vi "sharp_ir_long.vi"(11 "ana_volts":dbl) -> (3 "eng_cm":dbl)   [LabVIEW 2012]
panel:
  in  "cm":dbl[](array[numeric])=[200.0, 150.0, 140.0, 130.0, 120.0, 110.0, 100.0, 90.0, 80.0, 70.0, 60.0, 50.0, 40.0, 30.0, 20.0, 15.0, 0.0]
  in  "volts":dbl[](array[numeric])=[0.0, 0.4, 0.45, 0.5, 0.55, 0.6, 0.66, 0.73, 0.8, 0.86, 1.07, 1.25, 1.56, 2.0, 2.5, 2.75, 5.0]
  # "This function is a transfer function for the Sharp IR GP2Y0A02YK0F long range IR rangefinder\nThis curve is copied directly from the Sharp spec sheet transfer curve. Units are cm in that sheet."
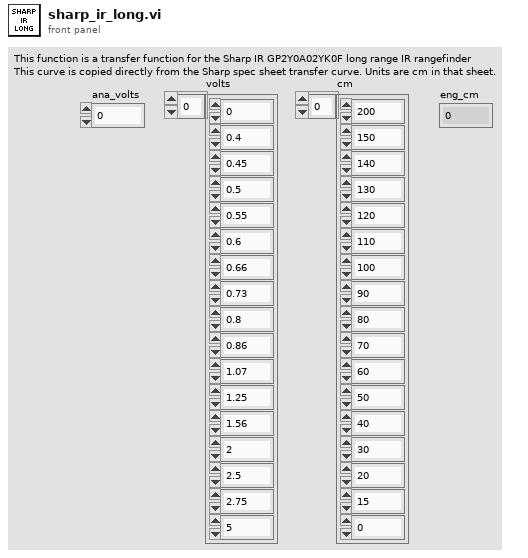
[diagram p1: front panel]
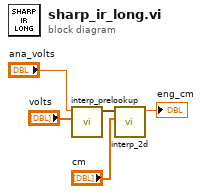
[diagram p0: block diagram]
diagram:
  n1 = call "interp_prelookup.vi"("x"="volts", "X"="ana_volts") -> ("prelookup"=w3:cluster{"frac":dbl, "num":u8})  [unwired: 8 in, 1 out]
  n2 = call "interp_2d.vi"("z"="cm", "prelookup"=w3) -> ("z"=→"eng_cm":dbl)  [unwired: 9 in]
